vi "Control Panel.vi"() -> ()   [LabVIEW 2018]
uses:
  <instrlib>/NHRDCPowerModule/NHRDCPowerModule/NHRDCPowerModule.lvlib
panel:
  in  "EVENT: Run macro":bool
  out "Current Macro":string
  in  "EVENT Load macro":bool
  out "Macro Dialog":string
  in  "EVENT Edit macro":bool
  out "Voltage Slew":sgl caption="Voltage" format="%#_3pV/s"
  out "Current Slew":sgl caption="Current" format="%#_3pA/s"
  out "Power Slew":sgl caption="Power" format="%#_3pW/s"
  out "Resistance Slew":sgl caption="Resistance" format="%#_3pOhm/s"
  in  "Set Resistance Slew":sgl caption="Resistance" format="%#_3pOhm/s"
  in  "Set Power Slew":sgl caption="Power" format="%#_3pW/s"
  in  "Set Current Slew":sgl caption="Current" format="%#_3pA/s"
  in  "Set Voltage Slew":sgl caption="Voltage" format="%#_3pV/s"
  in  "EVENT Set slew rates":bool
  in  "EVENT Reset":bool
  in  "EVENT Clear error":bool
  out "error message":string caption="Error Message"
  out "Resistance":sgl format="%#_3pOhm"
  out "Power":sgl format="%#_3pW"
  out "Current":sgl format="%#_3pA"
  out "Voltage":sgl format="%#_3pV"
  in  "Set Operating State":i32(ring)=2 caption="Operating State" items=["Off", "Stand By", "Charge", "Discharge", "Battery Emulation"]
  in  "EVENT Set state":bool
  in  "Set Resistance":sgl caption="Resistance" format="%#_3pOhm"
  in  "Set Resistance?":bool
  in  "Set Power":sgl caption="Power" format="%#_3pW"
  in  "Set Power?":bool
  in  "Set Current":sgl caption="Current" format="%#_3pA"
  in  "Set Current?":bool
  in  "Set Voltage":sgl caption="Voltage" format="%#_3pV"
  in  "Set Voltage?":bool
  in  "EVENT Set safety limits":bool
  in  "Set Voltage Safety Limit":sgl caption="Voltage" format="%#_3pV"
  in  "Set Voltage Delay Safety Limit":sgl caption="Voltage Delay" min=0 format="%#_3ps"
  in  "Set Current Delay Safety Limit":sgl caption="Current Delay" min=0 format="%#_3ps"
  in  "Set Current Safety Limit":sgl caption="Current" min=0 format="%#_3pA"
  in  "Set Power Delay Safety Limit":sgl caption="Power Delay" min=0 format="%#_3ps"
  in  "Set Power Safety Limit":sgl caption="Power" min=0 format="%#_3pW"
  out "Voltage Safety Limit":sgl caption="Voltage Max" format="%#_3pV"
  out "Voltage Delay Safety Limit":sgl caption="Voltage Delay" format="%#_3ps"
  out "Current Delay Safety Limit":sgl caption="Current Delay" format="%#_3ps"
  out "Current Safety Limit":sgl caption="Current" format="%#_3pA"
  out "Power Delay Safety Limit":sgl caption="Power Delay" format="%#_3ps"
  out "Power Safety Limit":sgl caption="Power" format="%#_3pW"
  in  "EVENT Safety Limit Type":enum16{"Charge", "Discharge"}(ring) caption="Limit Type"
  in  "EVENT Exit":bool
  # "add spectroscopy bits"
  # "enforce state dependent max/min values"
  # "Macro"
  # "Set Slew Rates"
  # "New"
  # "Current"
  # "Error"
  # "Set NHR State"
  # "Set?"
  # "New"
  # "Current"
  # "Set Safety Limits"
  # "New"
  # "Current"
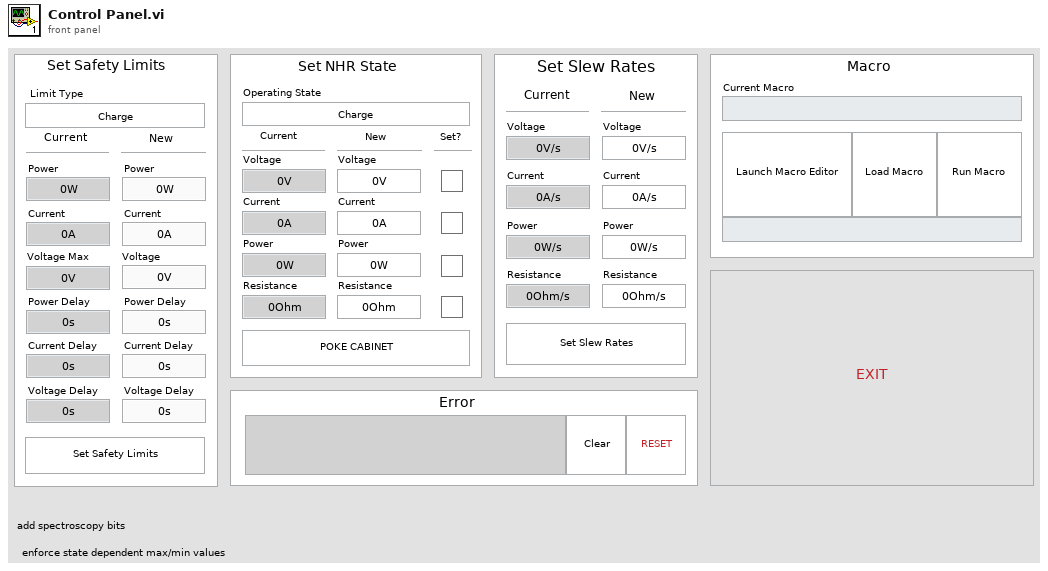
[diagram p1: front panel]
types:
  T1 = enum8{"Enabled", "Disabled", "Disabled and Grayed Out"}
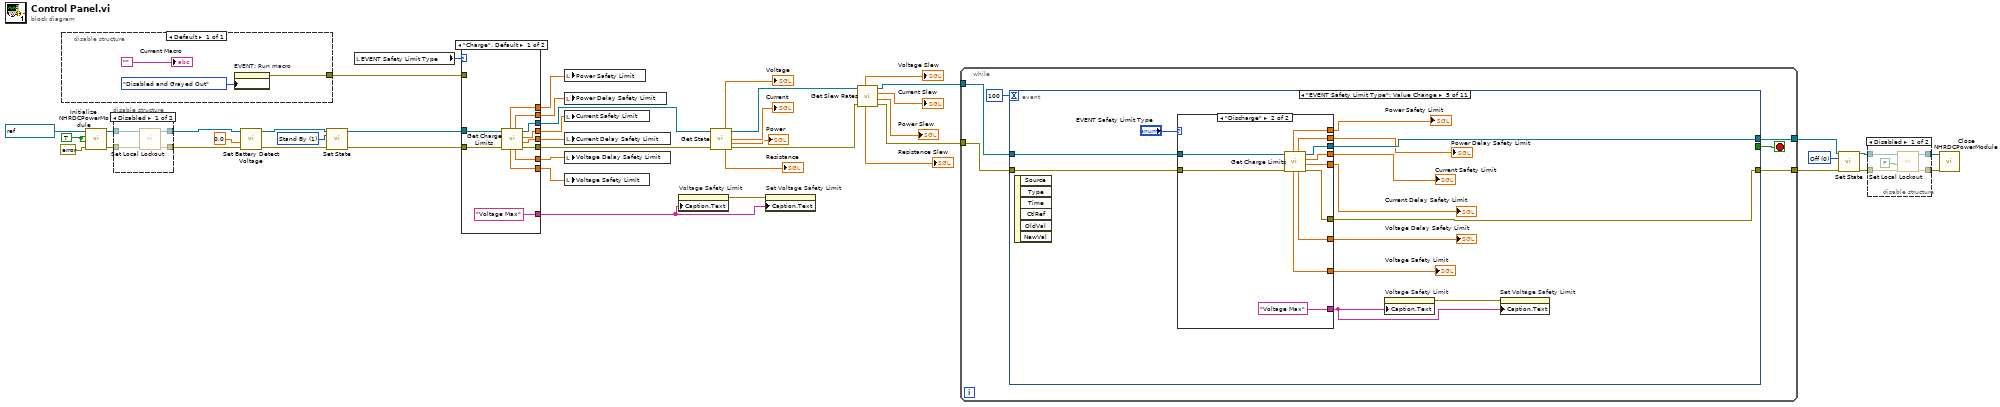
[diagram p0: block diagram]
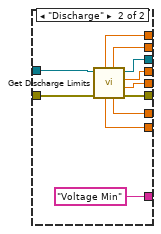
[diagram p2: hidden frame]
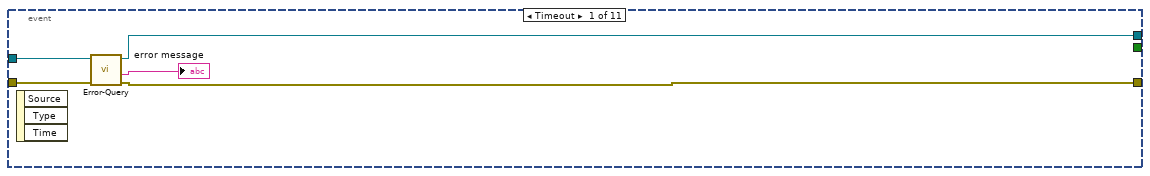
[diagram p5: hidden frame]
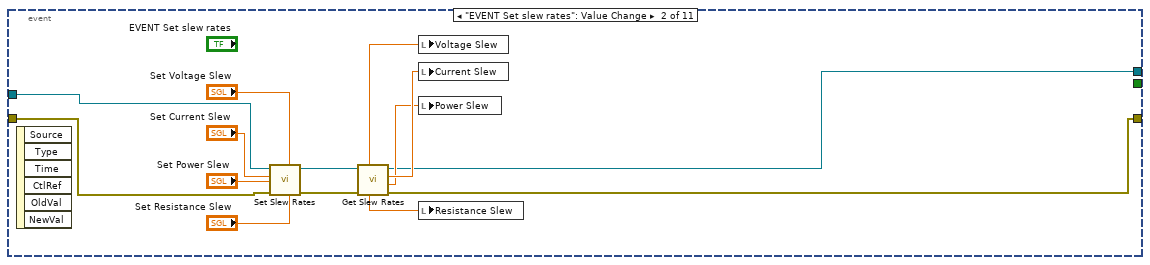
[diagram p6: hidden frame]
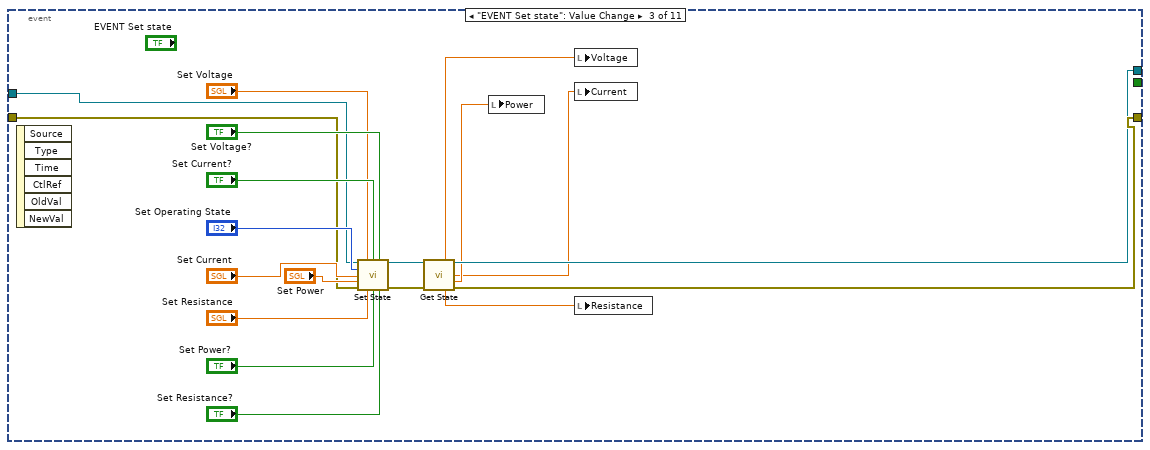
[diagram p7: hidden frame]
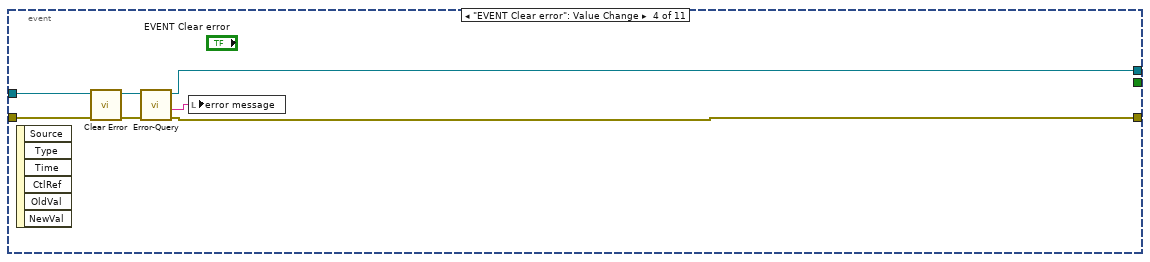
[diagram p8: hidden frame]
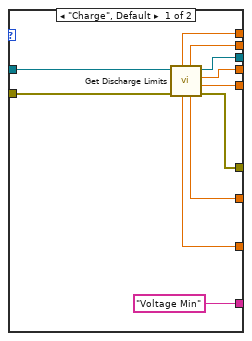
[diagram p9: hidden frame]
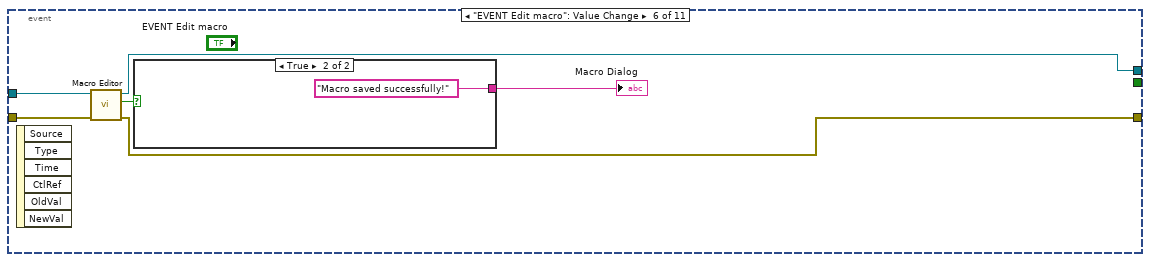
[diagram p10: hidden frame]
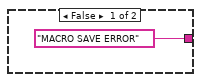
[diagram p11: hidden frame]
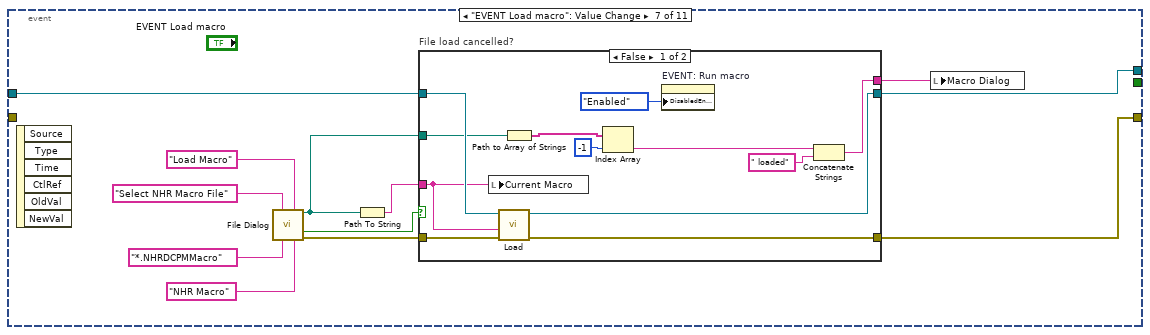
[diagram p12: hidden frame]
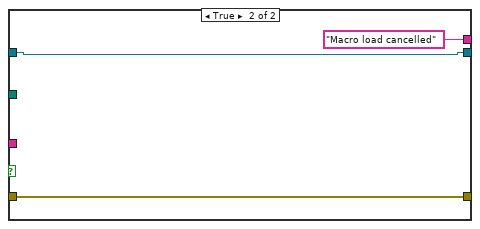
[diagram p13: hidden frame]
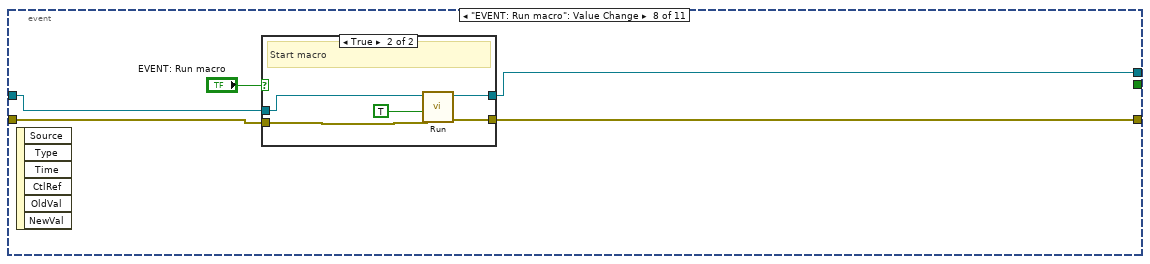
[diagram p14: hidden frame]
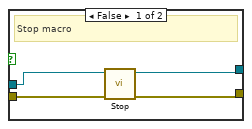
[diagram p15: hidden frame]
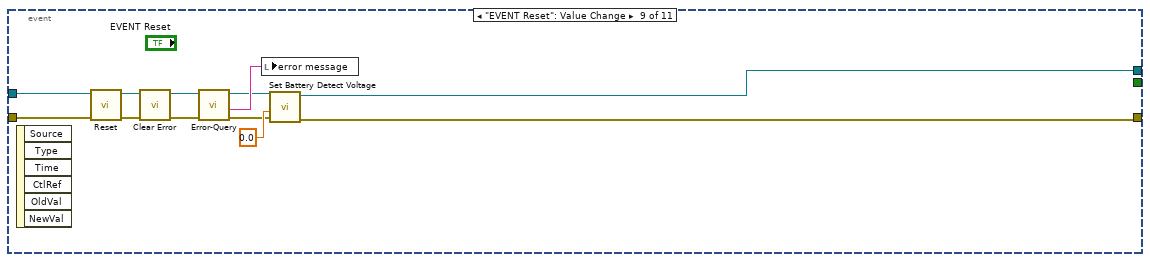
[diagram p16: hidden frame]
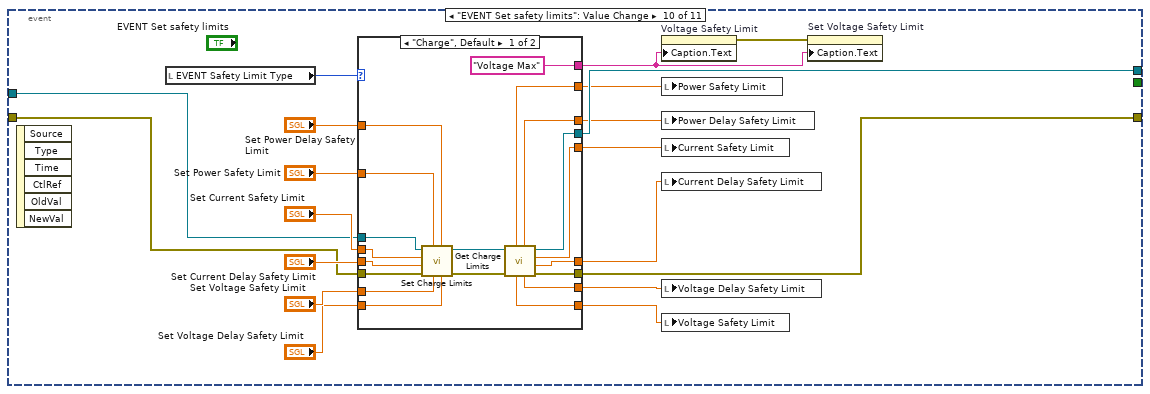
[diagram p17: hidden frame]
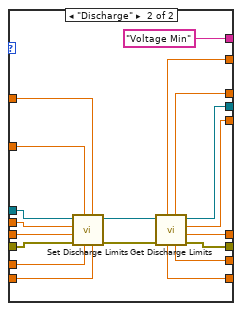
[diagram p18: hidden frame]
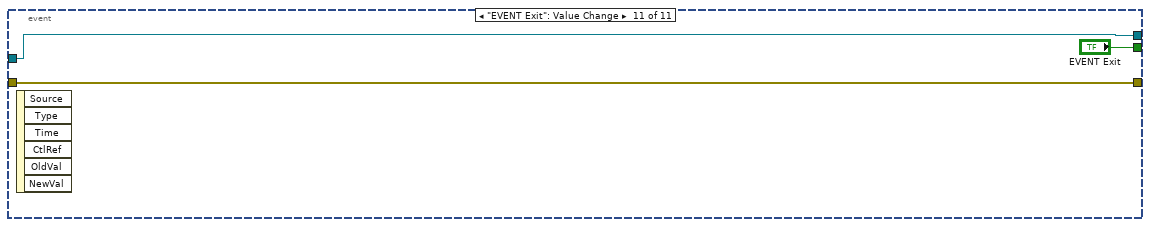
[diagram p19: hidden frame]
diagram:
  w37 = 0 items=["Off", "Stand By", "Charge", "Discharge", "Battery Emulation"] ("operating state (Off)")
  w38 = TRUE ("reset device (Off)")
  w41 = 1 items=["Off", "Stand By", "Charge", "Discharge", "Battery Emulation"] ("operating state (Off)")
  n1 = disable-structure shown="Default" {
    disable-tunnel: [w45] -> w1
    frame Enabled {
      n2 = property on="EVENT: Run macro" class="Bool (strict)"("DisabledEnum"=T1."Disabled and Grayed Out" ("Disabled")) -> (error out=w45:errorcluster)  [unwired: 2 in, 1 out]
      "Current Macro" <- ""
    }
  }
  n3 = call <instrlib>:"Initialize NHRDCPowerModule.vi"("error in (no error)"=errorcluster {"status"=FALSE, "code"=0, "source"=""}, "reset device (Off)"=w38, "id query (Off)"=w38, "resource name"=refnum<visa-resource-name> "DC PM 1" ("instrument handle")) -> ("error out"=w28:errorcluster, "instrument handle out"=w27:refnum<visa-resource-name>)  [unwired: 6 in]
  n4 = disable-structure shown="Disabled" {
    disable-tunnel: [w51 _] -> w30
    disable-tunnel: [w50 _] -> w29
    disable-tunnel: w28 -> [w49 _]
    disable-tunnel: w27 -> [w48 _]
    frame Disabled {
      n5 = call <instrlib>:"Set Local Lockout.vi"("error in (no error)"=w49, "instrument handle"=w48) -> ("error out"=w51:errorcluster, "instrument handle out"=w50:refnum<visa-resource-name>)  [unwired: 8 in]
    }
    frame Enabled {
    }
  }
  n6 = call <instrlib>:"Set Battery Detect Voltage.vi"("error in (no error)"=w30, "minimum voltage (4.0)"=sgl 0.0, "instrument handle"=w29) -> ("error out"=w42:errorcluster, "instrument handle out"=w43:refnum<visa-resource-name>)  [unwired: 7 in]
  n7 = call <instrlib>:"Set State.vi"("instrument handle"=w43, "operating state (Off)"=w41, "error in (no error)"=w42) -> ("instrument handle out"=w13:refnum<visa-resource-name>, "error out"=w11:errorcluster)  [unwired: 11 in]
  n8 = local read "EVENT Safety Limit Type"() -> (w14:enum16{"Charge", "Discharge"})
  n9 = case shown="\"Charge\", Default" w14 {
    tunnel: [w61 w72] -> w12
    tunnel: [w62 w73] -> w10
    tunnel: [w58 w66] -> w15
    tunnel: [w59 w65] -> w16
    tunnel: [w57 w71] -> w17
    tunnel: [w56 w70] -> w18
    tunnel: [w55 w69] -> w19
    tunnel: [w54 w68] -> w20
    tunnel: ["Voltage Max" ("Caption.Text") "Voltage Min" ("Caption.Text")] -> w21
    tunnel: w13 -> [w53 w64]
    tunnel: w11 -> [w52 w63]
    tunnel: w1 -> [_ _]
    frame "Charge", Default {
      n10 = call <instrlib>:"Get Charge Limits.vi"("error in (no error)"=w52, "instrument handle"=w53) -> ("error out"=w62:errorcluster, "current delay"=w56:sgl, "current"=w57:sgl, "instrument handle out"=w61:refnum<visa-resource-name>, "voltage delay"=w54:sgl, "power delay"=w59:sgl, "voltage max"=w55:sgl, "power"=w58:sgl)  [unwired: 2 in]
    }
    frame "Discharge" {
      n11 = call <instrlib>:"Get Discharge Limits.vi"("error in (no error)"=w63, "instrument handle"=w64) -> ("error out"=w73:errorcluster, "current delay"=w70:sgl, "current"=w71:sgl, "instrument handle out"=w72:refnum<visa-resource-name>, "voltage delay"=w68:sgl, "power delay"=w65:sgl, "voltage min"=w69:sgl, "power"=w66:sgl)  [unwired: 2 in]
    }
  }
  n12 = local write "Power Safety Limit"(w15) -> ()
  n13 = local write "Power Delay Safety Limit"(w16) -> ()
  n14 = local write "Current Safety Limit"(w17) -> ()
  n15 = local write "Current Delay Safety Limit"(w18) -> ()
  n16 = local write "Voltage Delay Safety Limit"(w20) -> ()
  n17 = local write "Voltage Safety Limit"(w19) -> ()
  n18 = property on="Voltage Safety Limit" class="DigNum (strict)"("Caption.Text"=w21) -> (error out=w22:errorcluster)  [unwired: 2 in, 1 out]
  n19 = call <instrlib>:"Get State.vi"("instrument handle"=w12, "error in (no error)"=w10) -> ("voltage"=→"Voltage":sgl, "instrument handle out"=w9:refnum<visa-resource-name>, "current"=→"Current":sgl, "power"=→"Power":sgl, "resistance"=→"Resistance":sgl, "error out"=w7:errorcluster)  [unwired: 3 in, 5 out]
  n20 = property on="Set Voltage Safety Limit" class="DigNum (strict)"(error in=w22, "Caption.Text"=w21) -> ()  [unwired: 1 in, 2 out]
  n21 = call "Get Slew Rates.vi"("error in (no error)"=w7, "instrument handle"=w9) -> ("error out"=w6:errorcluster, "power slew rate"=→"Power Slew":sgl, "current slew rate"=→"Current Slew":sgl, "instrument handle out"=w8:refnum<visa-resource-name>, "resistance slew rate"=→"Resistance Slew":sgl, "voltage slew rate"=→"Voltage Slew":sgl)  [unwired: 2 in]
  n22 = while {
    tunnel: w8 -> [w78]
    tunnel: w6 -> [w77]
    tunnel: [w76] -> w36
    tunnel: [w75] -> w35
    stop <- w79 stop-if-true
    n23 = event shown="[4] \"EVENT Safety Limit Type\": Value Change" {
      selector: _ -> [_ _ _ _ _ _ _ _ _ _ _]
      dyn-events: _ -> [_ _ _ _ _ _ _ _ _ _ _]
      timeout: 100 -> [_ _ _ _ _ _ _ _ _ _ _]
      tunnel: [_ _ _ _ _ _ _ _ _ _ "EVENT Exit"] -> w79
      tunnel: w78 -> [w84 w96 w108 w118 w136 w165 w172 w198 w219 w232 w279]
      tunnel: w77 -> [w83 w95 w107 w119 w135 w164 _ w197 w218 w231 w278]
      tunnel: [w80 w85 w103 w123 w134 w162 w171 w196 w209 w230 w279] -> w76
      tunnel: [w81 w86 w105 w122 w133 w163 w170 w195 w210 w229 w278] -> w75
      event Timeout {
        n24 = event-data() -> ()  [unwired: 1 in, 3 out]
        n25 = call <instrlib>:"Error-Query.vi"("error in (no error)"=w83, "instrument handle"=w84) -> ("error out"=w81:errorcluster, "error message"=→"error message":string, "instrument handle out"=w80:refnum<visa-resource-name>)  [unwired: 6 in, 1 out]
      }
      event "EVENT Set slew rates": Value Change {
        n26 = event-data() -> ()  [unwired: 1 in, 6 out]
        n27 = call "Set Slew Rates.vi"("instrument handle"=w96, "current slew rate"="Set Current Slew", "power slew rate"="Set Power Slew", "error in (no error)"=w95, "voltage slew rate"="Set Voltage Slew", "resistance slew rate"="Set Resistance Slew") -> ("instrument handle out"=w98:refnum<visa-resource-name>, "error out"=w97:errorcluster)  [unwired: 2 in]
        n28 = call "Get Slew Rates.vi"("error in (no error)"=w97, "instrument handle"=w98) -> ("error out"=w86:errorcluster, "power slew rate"=w88:sgl, "current slew rate"=w89:sgl, "instrument handle out"=w85:refnum<visa-resource-name>, "resistance slew rate"=w87:sgl, "voltage slew rate"=w90:sgl)  [unwired: 2 in]
        n29 = local write "Voltage Slew"(w90) -> ()
        n30 = local write "Current Slew"(w89) -> ()
        n31 = local write "Power Slew"(w88) -> ()
        n32 = local write "Resistance Slew"(w87) -> ()
      }
      event "EVENT Set state": Value Change {
        n33 = event-data() -> ()  [unwired: 1 in, 6 out]
        n34 = call <instrlib>:"Set State.vi"("instrument handle"=w108, "voltage (0.0)"="Set Voltage", "current enabled (false)"="Set Current?", "voltage enabled (false)"="Set Voltage?", "operating state (Off)"="Set Operating State", "current (0.0)"="Set Current", "power (0.0)"="Set Power", "error in (no error)"=w107, "resistance (0.0)"="Set Resistance", "power enabled (false)"="Set Power?", "resistance enabled (false)"="Set Resistance?") -> ("instrument handle out"=w104:refnum<visa-resource-name>, "error out"=w106:errorcluster)  [unwired: 3 in]
        n35 = call <instrlib>:"Get State.vi"("instrument handle"=w104, "error in (no error)"=w106) -> ("voltage"=w99:sgl, "instrument handle out"=w103:refnum<visa-resource-name>, "current"=w100:sgl, "power"=w101:sgl, "resistance"=w102:sgl, "error out"=w105:errorcluster)  [unwired: 3 in, 5 out]
        n36 = local write "Power"(w101) -> ()
        n37 = local write "Voltage"(w99) -> ()
        n38 = local write "Current"(w100) -> ()
        n39 = local write "Resistance"(w102) -> ()
      }
      event "EVENT Clear error": Value Change {
        n40 = event-data() -> ()  [unwired: 1 in, 6 out]
        n41 = call <instrlib>:"Clear Error.vi"("error in (no error)"=w119, "instrument handle"=w118) -> ("error out"=w120:errorcluster, "instrument handle out"=w121:refnum<visa-resource-name>)  [unwired: 8 in]
        n42 = call <instrlib>:"Error-Query.vi"("error in (no error)"=w120, "instrument handle"=w121) -> ("error out"=w122:errorcluster, "error message"=w124:string, "instrument handle out"=w123:refnum<visa-resource-name>)  [unwired: 6 in, 1 out]
        n43 = local write "error message"(w124) -> ()
      }
      event "EVENT Safety Limit Type": Value Change {
        n44 = event-data() -> ()  [unwired: 1 in, 6 out]
        n45 = case shown="\"Discharge\"" "EVENT Safety Limit Type" {
          tunnel: w136 -> [w147 w159]
          tunnel: w135 -> [w148 w158]
          tunnel: [w145 w157] -> w134
          tunnel: [w146 w150] -> w133
          tunnel: [w144 w156] -> w132
          tunnel: [w143 w155] -> w131
          tunnel: [w142 w154] -> w130
          tunnel: [w141 w153] -> w129
          tunnel: [w140 w152] -> w128
          tunnel: [w139 w151] -> w127
          tunnel: ["Voltage Min" ("Caption.Text") "Voltage Max" ("Caption.Text")] -> w126
          frame "Charge", Default {
            n46 = call <instrlib>:"Get Discharge Limits.vi"("error in (no error)"=w148, "instrument handle"=w147) -> ("error out"=w146:errorcluster, "current delay"=w141:sgl, "current"=w142:sgl, "instrument handle out"=w145:refnum<visa-resource-name>, "voltage delay"=w140:sgl, "power delay"=w143:sgl, "voltage min"=w139:sgl, "power"=w144:sgl)  [unwired: 2 in]
          }
          frame "Discharge" {
            n47 = call <instrlib>:"Get Charge Limits.vi"("error in (no error)"=w158, "instrument handle"=w159) -> ("error out"=w150:errorcluster, "current delay"=w153:sgl, "current"=w154:sgl, "instrument handle out"=w157:refnum<visa-resource-name>, "voltage delay"=w152:sgl, "power delay"=w155:sgl, "voltage max"=w151:sgl, "power"=w156:sgl)  [unwired: 2 in]
          }
        }
        "Power Safety Limit" <- w132
        "Power Delay Safety Limit" <- w131
        "Current Safety Limit" <- w130
        "Current Delay Safety Limit" <- w129
        "Voltage Delay Safety Limit" <- w128
        "Voltage Safety Limit" <- w127
        n48 = property on="Voltage Safety Limit" class="DigNum (strict)"("Caption.Text"=w126) -> (error out=w125:errorcluster)  [unwired: 2 in, 1 out]
        n49 = property on="Set Voltage Safety Limit" class="DigNum (strict)"(error in=w125, "Caption.Text"=w126) -> ()  [unwired: 1 in, 2 out]
      }
      event "EVENT Edit macro": Value Change {
        n50 = event-data() -> ()  [unwired: 1 in, 6 out]
        n51 = call <instrlib>:"Macro Editor.vi"("error in (no error)"=w164, "instrument handle"=w165) -> ("error out"=w163:errorcluster, "OK"=w161:bool, "instrument handle out"=w162:refnum<visa-resource-name>)  [unwired: 7 in]
        n52 = case shown="True" w161 {
          tunnel: ["MACRO SAVE ERROR" "Macro saved successfully!"] -> w160
          frame False {
          }
          frame True {
          }
        }
        "Macro Dialog" <- w160
      }
      event "EVENT Load macro": Value Change {
        n53 = event-data() -> ()  [unwired: 1 in, 6 out]
        n54 = call "File Dialog"("prompt"="Select NHR Macro File", "button label"="Load Macro", "pattern (all files)"="*.NHRDCPMMacro", "pattern label"="NHR Macro") -> ("selected path"=w169:path, "cancelled"=w175:bool, "error out"=w173:errorcluster)  [unwired: 8 in, 1 out]
        n55 = Path To String(path=w169) -> (string=w174:string)
        n56 = case "File load cancelled?" shown="False" w175 {
          tunnel: w174 -> [w189 _]
          tunnel: w173 -> [w191 w193]
          tunnel: w172 -> [w190 w194]
          tunnel: [w188 w194] -> w171
          tunnel: [w187 w193] -> w170
          tunnel: w169 -> [w181 _]
          tunnel: [w180 "Macro load cancelled"] -> w168
          frame False {
            n57 = local write "Current Macro"(w189) -> ()
            n58 = call <instrlib>:"Load.vi"("error in (no error)"=w191, "path (\"\")"=w189, "instrument handle"=w190) -> ("error out"=w187:errorcluster, "instrument handle out"=w188:refnum<visa-resource-name>)  [unwired: 7 in]
            n59 = Path to Array of Strings(0:w181) -> (2:w185:string[])  [unwired: 1 out]
            n60 = Index Array(array=w185, index=-1) -> (element=w184:string)
            n61 = property on="EVENT: Run macro" class="Bool (strict)"("DisabledEnum"=T1."Enabled" ("Disabled")) -> ()  [unwired: 2 in, 2 out]
            n62 = Concatenate Strings(w184, " loaded") -> (w180:string)
          }
          frame True {
          }
        }
        n63 = local write "Macro Dialog"(w168) -> ()
      }
      event "EVENT: Run macro": Value Change {
        n64 = event-data() -> ()  [unwired: 1 in, 6 out]
        n65 = case shown="True" "EVENT: Run macro" {
          tunnel: w198 -> [w203 w207]
          tunnel: w197 -> [w202 w206]
          tunnel: [w200 w205] -> w196
          tunnel: [w201 w204] -> w195
          frame False {
            # "Stop macro"
            n66 = call <instrlib>:"Stop.vi"("error in (no error)"=w202, "instrument handle"=w203) -> ("error out"=w201:errorcluster, "instrument handle out"=w200:refnum<visa-resource-name>)  [unwired: 8 in]
          }
          frame True {
            # "Start macro"
            n67 = call <instrlib>:"Run.vi"("error in (no error)"=w206, "continuous (false)"=TRUE, "instrument handle"=w207) -> ("error out"=w204:errorcluster, "instrument handle out"=w205:refnum<visa-resource-name>)  [unwired: 7 in]
          }
        }
      }
      event "EVENT Reset": Value Change {
        n68 = event-data() -> ()  [unwired: 1 in, 6 out]
        n69 = call <instrlib>:"Reset.vi"("error in (no error)"=w218, "instrument handle"=w219) -> ("error out"=w216:errorcluster, "instrument handle out"=w217:refnum<visa-resource-name>)  [unwired: 8 in]
        n70 = call <instrlib>:"Clear Error.vi"("error in (no error)"=w216, "instrument handle"=w217) -> ("error out"=w215:errorcluster, "instrument handle out"=w214:refnum<visa-resource-name>)  [unwired: 8 in]
        n71 = call <instrlib>:"Error-Query.vi"("error in (no error)"=w215, "instrument handle"=w214) -> ("error out"=w211:errorcluster, "error message"=w220:string, "instrument handle out"=w212:refnum<visa-resource-name>)  [unwired: 6 in, 1 out]
        n72 = local write "error message"(w220) -> ()
        n73 = call <instrlib>:"Set Battery Detect Voltage.vi"("error in (no error)"=w211, "minimum voltage (4.0)"=sgl 0.0, "instrument handle"=w212) -> ("error out"=w210:errorcluster, "instrument handle out"=w209:refnum<visa-resource-name>)  [unwired: 7 in]
      }
      event "EVENT Set safety limits": Value Change {
        n74 = event-data() -> ()  [unwired: 1 in, 6 out]
        n75 = local read "EVENT Safety Limit Type"() -> (w239:enum16{"Charge", "Discharge"})
        n76 = case shown="\"Charge\", Default" w239 {
          tunnel: "Set Current Safety Limit" -> [w255 w277]
          tunnel: "Set Current Delay Safety Limit" -> [w256 w276]
          tunnel: "Set Power Safety Limit" -> [w254 w275]
          tunnel: "Set Voltage Safety Limit" -> [w241 w274]
          tunnel: "Set Voltage Delay Safety Limit" -> [w240 w273]
          tunnel: "Set Power Delay Safety Limit" -> [w253 w272]
          tunnel: w232 -> [w258 w271]
          tunnel: w231 -> [w257 w270]
          tunnel: [w249 w266] -> w230
          tunnel: [w250 w267] -> w229
          tunnel: [w246 w260] -> w228
          tunnel: [w247 w259] -> w227
          tunnel: [w245 w265] -> w226
          tunnel: [w244 w264] -> w225
          tunnel: [w243 w263] -> w224
          tunnel: [w242 w262] -> w223
          tunnel: ["Voltage Max" ("Caption.Text") "Voltage Min" ("Caption.Text")] -> w222
          frame "Charge", Default {
            n77 = call <instrlib>:"Set Charge Limits.vi"("voltage delay (0.0)"=w240, "power delay (0.0)"=w253, "voltage max"=w241, "power"=w254, "error in (no error)"=w257, "current delay (0.0)"=w256, "current"=w255, "instrument handle"=w258) -> ("error out"=w251:errorcluster, "instrument handle out"=w252:refnum<visa-resource-name>)  [unwired: 2 in]
            n78 = call <instrlib>:"Get Charge Limits.vi"("error in (no error)"=w251, "instrument handle"=w252) -> ("error out"=w250:errorcluster, "current delay"=w244:sgl, "current"=w245:sgl, "instrument handle out"=w249:refnum<visa-resource-name>, "voltage delay"=w242:sgl, "power delay"=w247:sgl, "voltage max"=w243:sgl, "power"=w246:sgl)  [unwired: 2 in]
          }
          frame "Discharge" {
            n79 = call <instrlib>:"Set Discharge Limits.vi"("voltage delay (0.0)"=w273, "power delay (0.0)"=w272, "voltage min"=w274, "power"=w275, "error in (no error)"=w270, "current delay (0.0)"=w276, "current"=w277, "instrument handle"=w271) -> ("error out"=w268:errorcluster, "instrument handle out"=w269:refnum<visa-resource-name>)  [unwired: 2 in]
            n80 = call <instrlib>:"Get Discharge Limits.vi"("error in (no error)"=w268, "instrument handle"=w269) -> ("error out"=w267:errorcluster, "current delay"=w264:sgl, "current"=w265:sgl, "instrument handle out"=w266:refnum<visa-resource-name>, "voltage delay"=w262:sgl, "power delay"=w259:sgl, "voltage min"=w263:sgl, "power"=w260:sgl)  [unwired: 2 in]
          }
        }
        n81 = property on="Voltage Safety Limit" class="DigNum (strict)"("Caption.Text"=w222) -> (error out=w221:errorcluster)  [unwired: 2 in, 1 out]
        n82 = local write "Power Safety Limit"(w228) -> ()
        n83 = local write "Power Delay Safety Limit"(w227) -> ()
        n84 = local write "Current Safety Limit"(w226) -> ()
        n85 = local write "Current Delay Safety Limit"(w225) -> ()
        n86 = local write "Voltage Delay Safety Limit"(w223) -> ()
        n87 = local write "Voltage Safety Limit"(w224) -> ()
        n88 = property on="Set Voltage Safety Limit" class="DigNum (strict)"(error in=w221, "Caption.Text"=w222) -> ()  [unwired: 1 in, 2 out]
      }
      event "EVENT Exit": Value Change {
        n89 = event-data() -> ()  [unwired: 1 in, 6 out]
      }
    }
  }
  n90 = call <instrlib>:"Set State.vi"("instrument handle"=w36, "operating state (Off)"=w37, "error in (no error)"=w35) -> ("instrument handle out"=w25:refnum<visa-resource-name>, "error out"=w26:errorcluster)  [unwired: 11 in]
  n91 = disable-structure shown="Disabled" {
    disable-tunnel: w26 -> [w284 _]
    disable-tunnel: w25 -> [w283 _]
    disable-tunnel: [w282 _] -> w24
    disable-tunnel: [w281 _] -> w23
    frame Disabled {
      n92 = call <instrlib>:"Set Local Lockout.vi"("error in (no error)"=w284, "locked (true)"=FALSE, "instrument handle"=w283) -> ("error out"=w281:errorcluster, "instrument handle out"=w282:refnum<visa-resource-name>)  [unwired: 7 in]
    }
    frame Enabled {
    }
  }
  n93 = call <instrlib>:"Close NHRDCPowerModule.vi"("error in (no error)"=w23, "instrument handle"=w24) -> ()  [unwired: 9 in, 1 out]
